vi "Parse Controls Log.vi"(8 "error in (no error)":errorcluster, 11 "Controls Log File":path) -> (0 "error out":errorcluster, 3 "Parsed Pulse Data":T1(array[cluster]))   [LabVIEW 2013, in "Controls Log Monitor.lvlib"]
uses:
  ControlLogParserStateMachineStates.ctl
  PulseData.lvclass
  <vilib>/Utility/miscctls.llb/LVDateTimeRec.ctl
  <vilib>/Utility/file.llb/Read From Spreadsheet File (string).vi
  Controls Log Monitor.lvlib
panel:
  out "Line After Comment":string
  out "Pulse Data Cluster":T2
  out "Entry Index":i32
  out "Pulse Count":i32
  out "Run #":i32
  out "size(s)":i32[](array[numeric])
  out "all rows":string[][](array[string])
  # "68625"
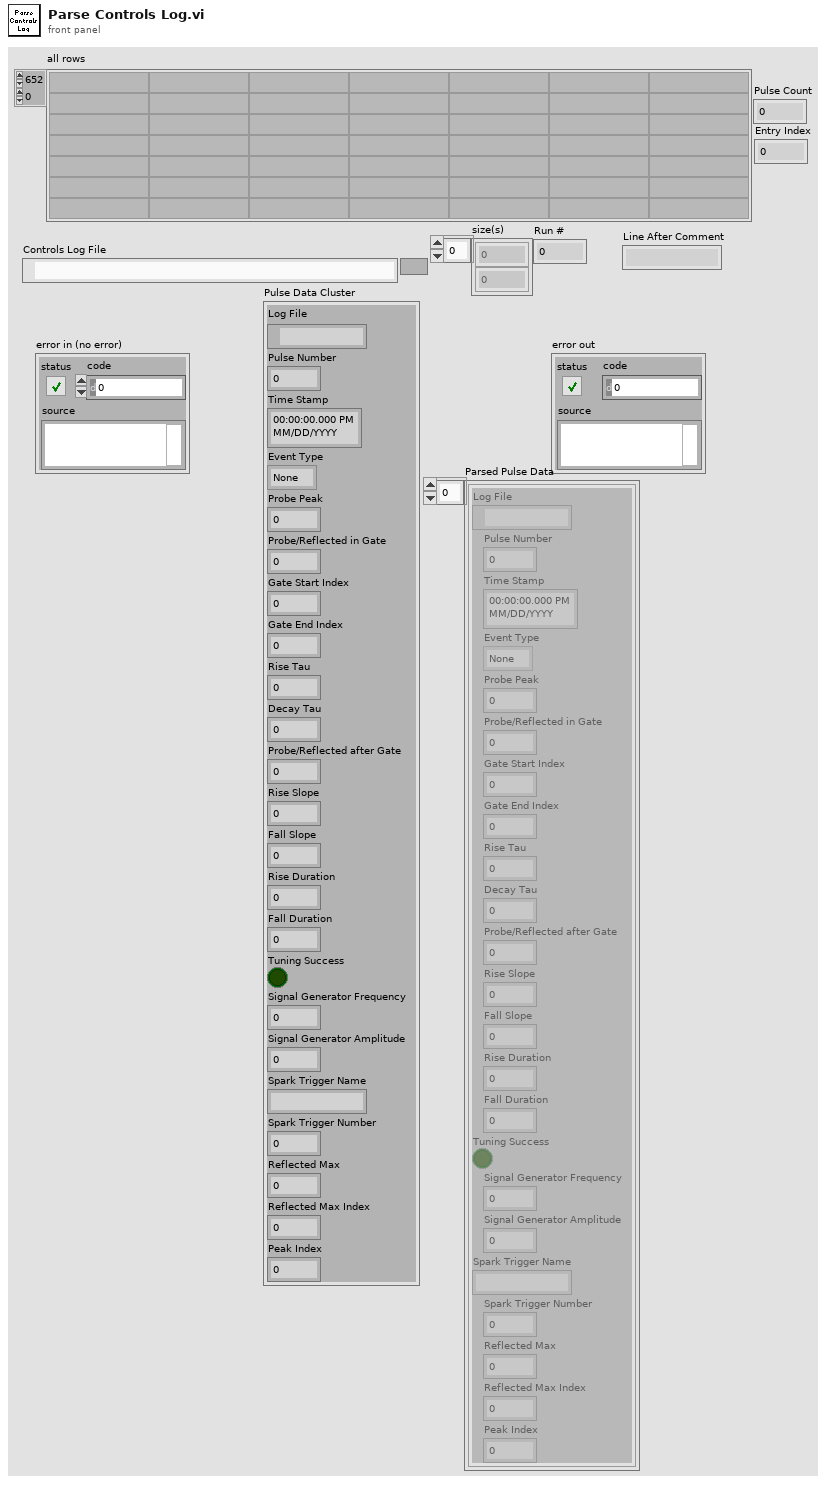
[diagram p1: front panel]
types:
  T1 = cluster{"Log File":path, "Pulse Number":u32, "Time Stamp":timestamp, "Event Type":enum16{"None", "Tune", "Periodic Capture", "Spark Trigger"}, "Probe Peak":dbl, "Probe/Reflected in Gate":dbl, "Gate Start Index":i32, "Gate End Index":i32, "Rise Tau":dbl, "Decay Tau":dbl, "Probe/Reflected after Gate":dbl, "Rise Slope":dbl, "Fall Slope":dbl, "Rise Duration":dbl, "Fall Duration":dbl, "Tuning Success":bool, "Signal Generator Frequency":dbl, "Signal Generator Amplitude":dbl, "Spark Trigger Name":string, "Spark Trigger Number":i32, "Reflected Max":dbl, "Reflected Max Index":i32, "Peak Index":i32}[]
  T2 = cluster{"Log File":path, "Pulse Number":u32, "Time Stamp":timestamp, "Event Type":enum16{"None", "Tune", "Periodic Capture", "Spark Trigger"}, "Probe Peak":dbl, "Probe/Reflected in Gate":dbl, "Gate Start Index":i32, "Gate End Index":i32, "Rise Tau":dbl, "Decay Tau":dbl, "Probe/Reflected after Gate":dbl, "Rise Slope":dbl, "Fall Slope":dbl, "Rise Duration":dbl, "Fall Duration":dbl, "Tuning Success":bool, "Signal Generator Frequency":dbl, "Signal Generator Amplitude":dbl, "Spark Trigger Name":string, "Spark Trigger Number":i32, "Reflected Max":dbl, "Reflected Max Index":i32, "Peak Index":i32}
  T3 = typedef "ControlLogParserStateMachineStates.ctl" = enum16{"Load Log", "Initialize Pulse", "Parse Pulse", "Parse Comment", "Finalize Pulse", "Stop", ""}
  T4 = typedef "LVDateTimeRec.ctl" = cluster{"fractional second":dbl, "second":i32, "minute":i32, "hour":i32, "day of month":i32, "month":i32, "year":i32, "day of week":i32, "day of year":i32, "DST":i32}
  T5 = enum16{"None", "Tune", "Periodic Capture", "Spark Trigger"}
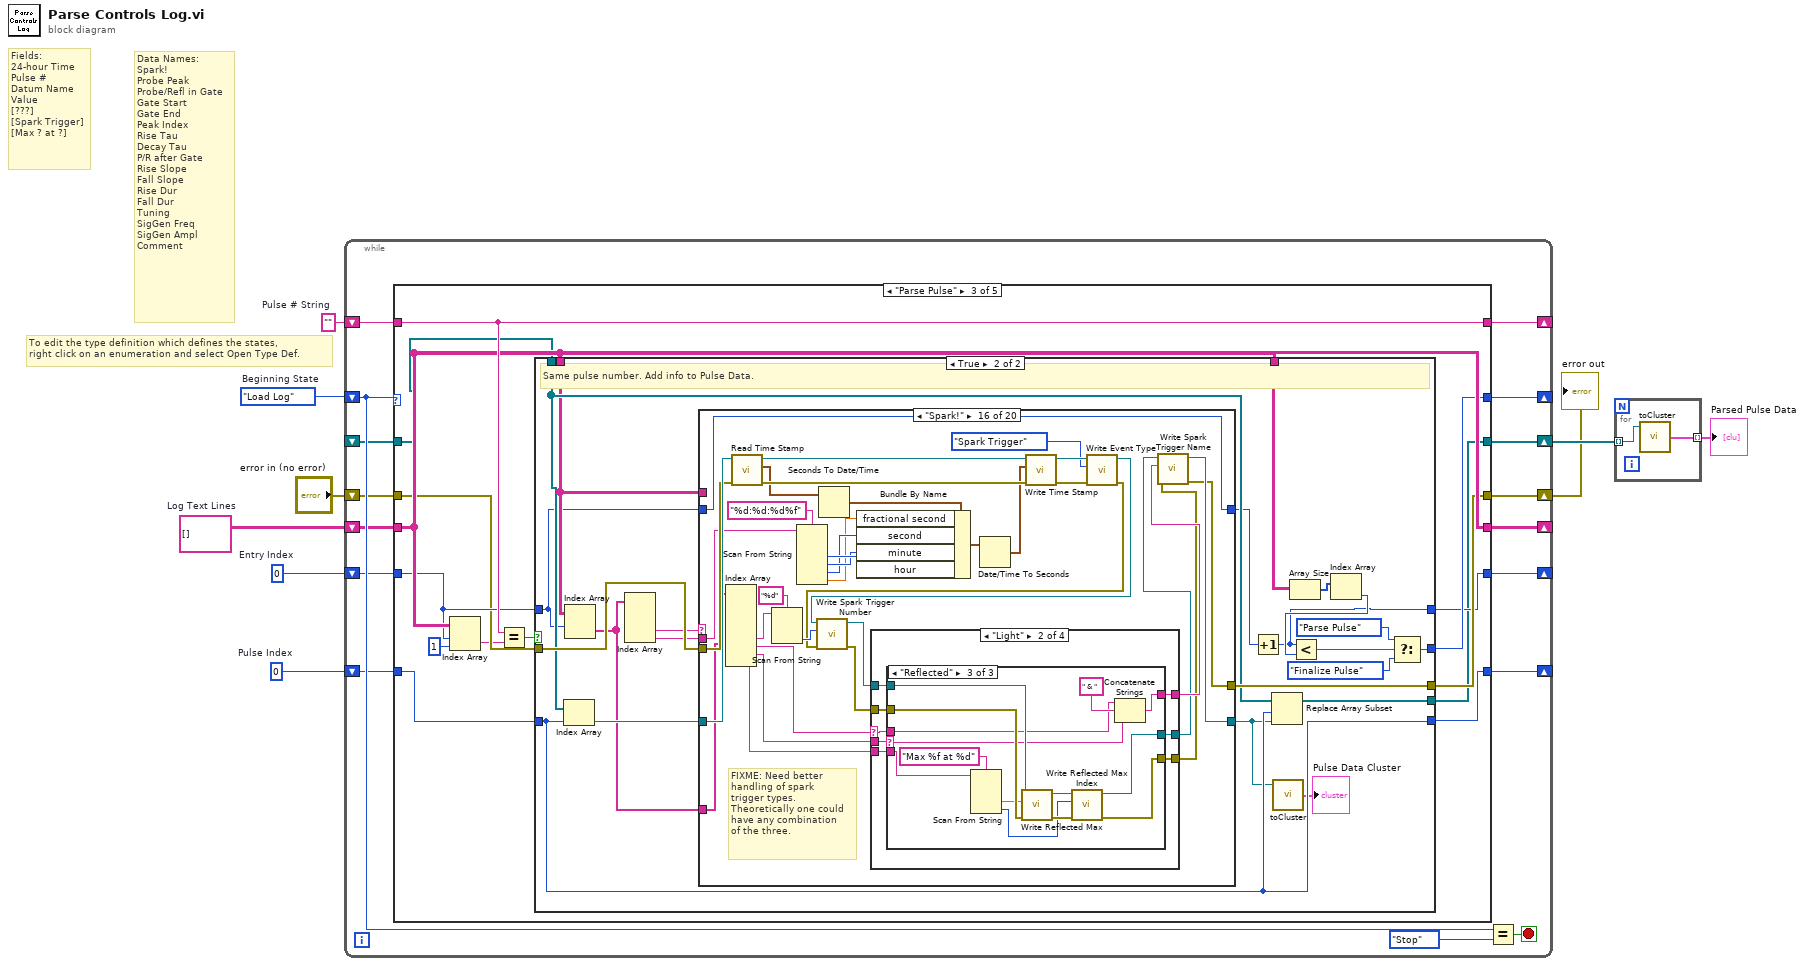
[diagram p0: block diagram]
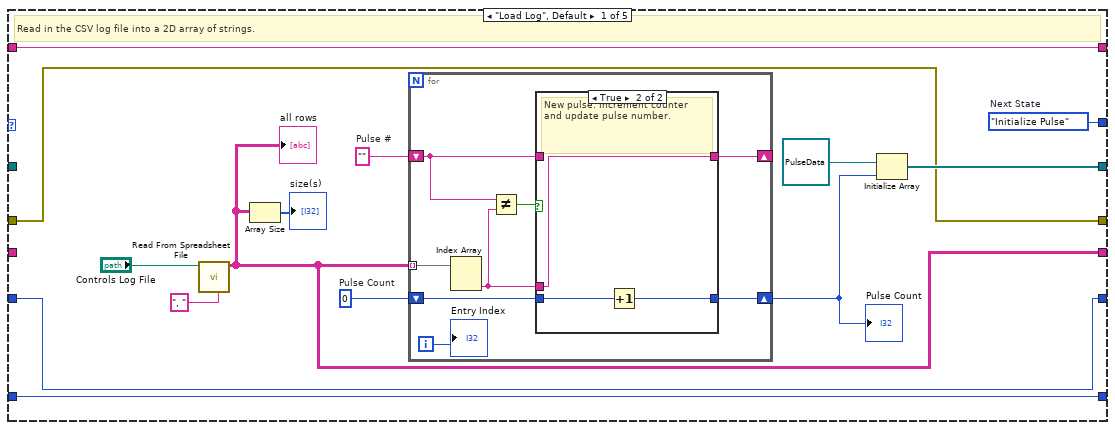
[diagram p2: hidden frame]
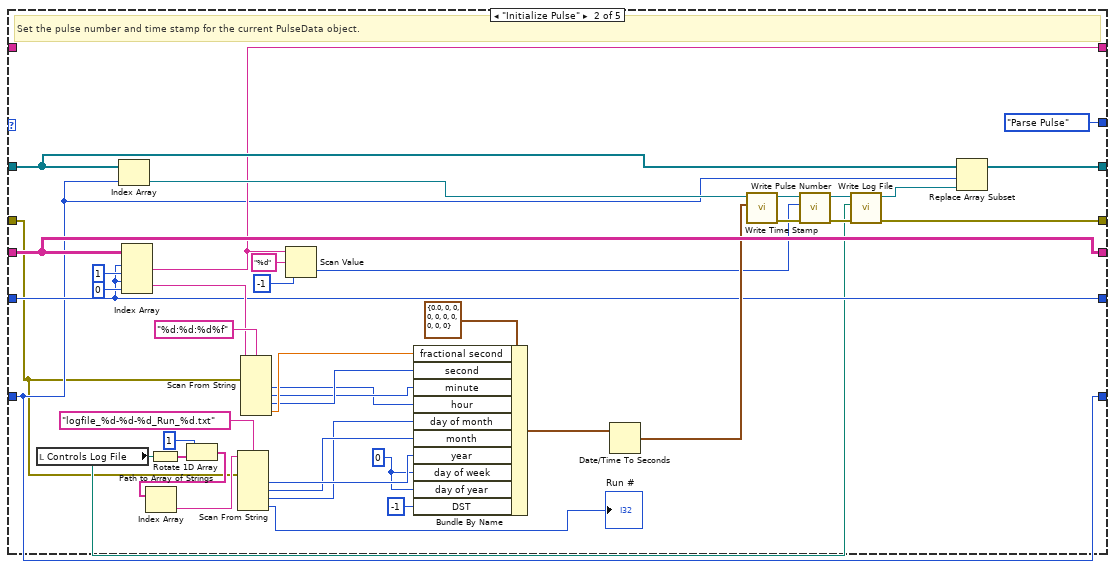
[diagram p4: hidden frame]
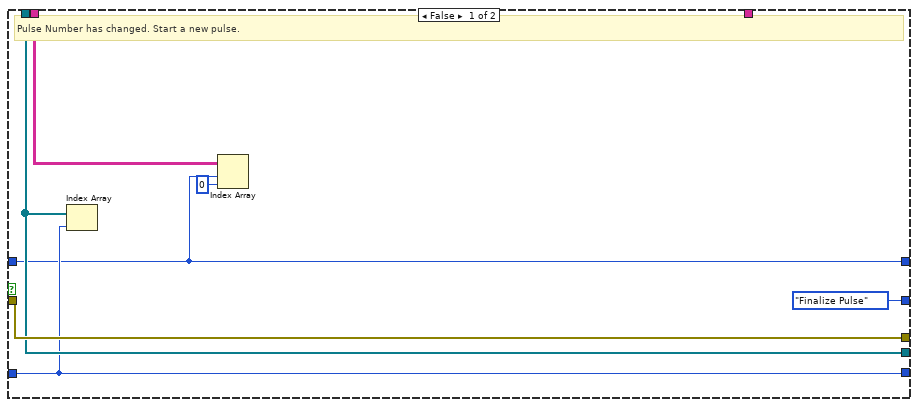
[diagram p5: hidden frame]
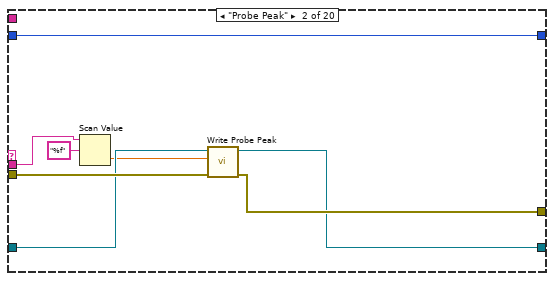
[diagram p7: hidden frame]
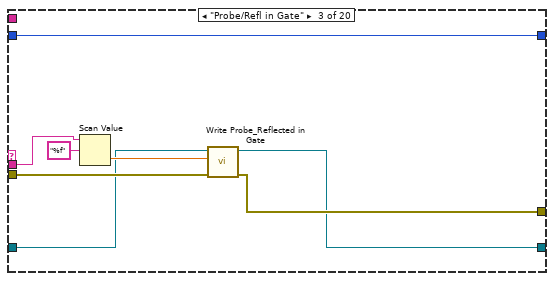
[diagram p8: hidden frame]
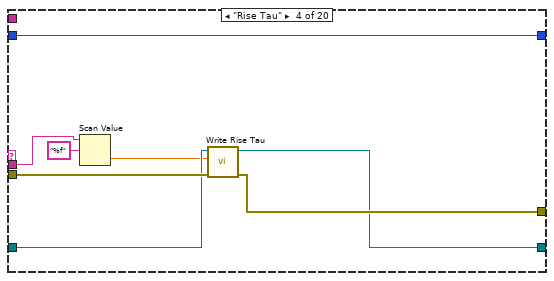
[diagram p9: hidden frame]
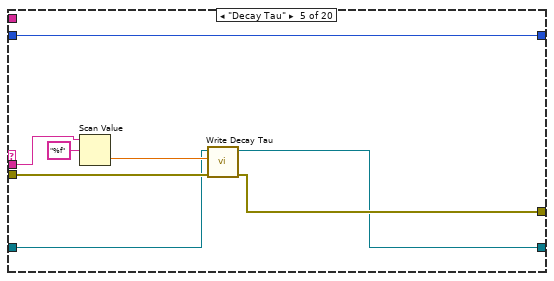
[diagram p10: hidden frame]
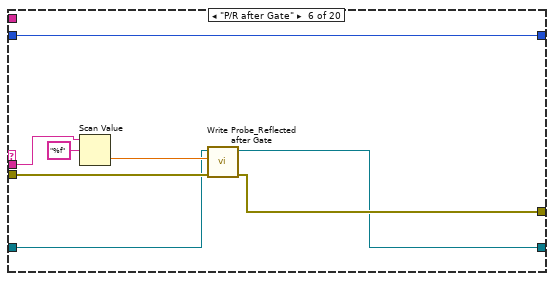
[diagram p11: hidden frame]
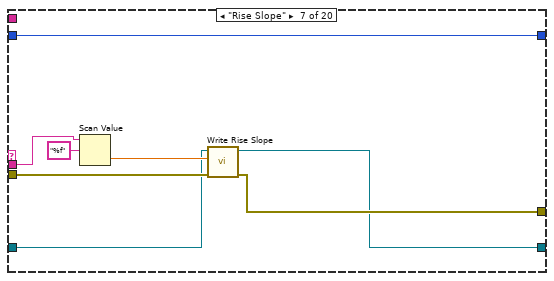
[diagram p12: hidden frame]
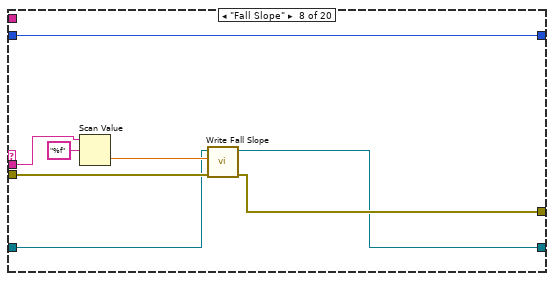
[diagram p13: hidden frame]
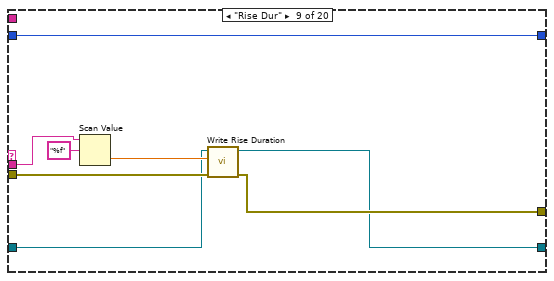
[diagram p14: hidden frame]
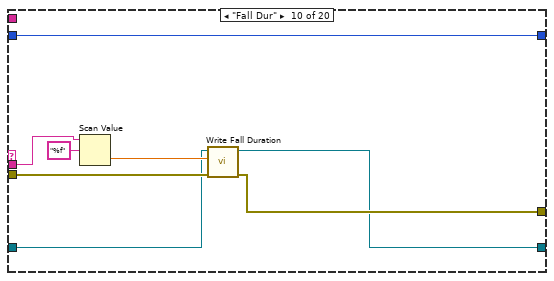
[diagram p15: hidden frame]
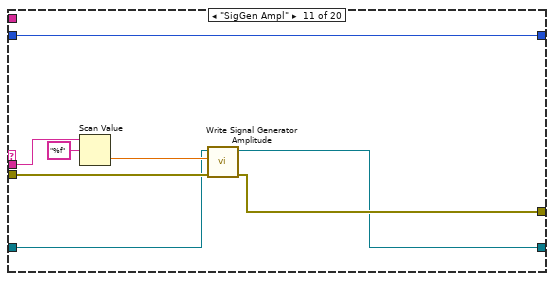
[diagram p16: hidden frame]
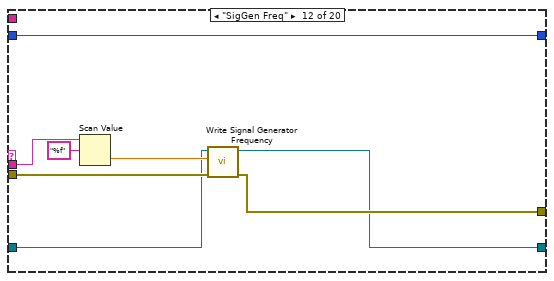
[diagram p17: hidden frame]
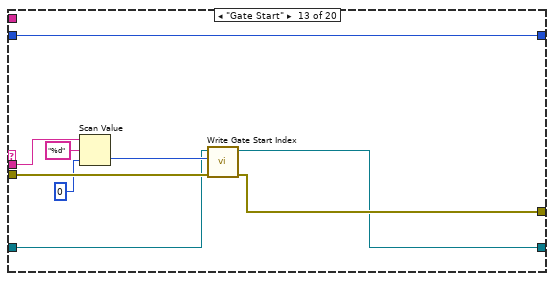
[diagram p18: hidden frame]
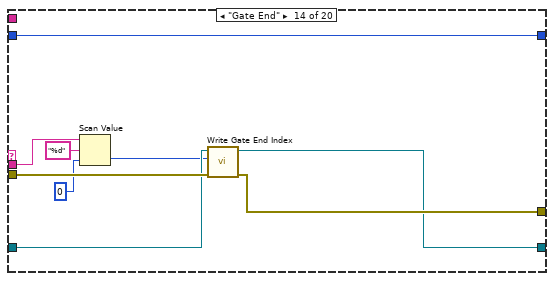
[diagram p19: hidden frame]
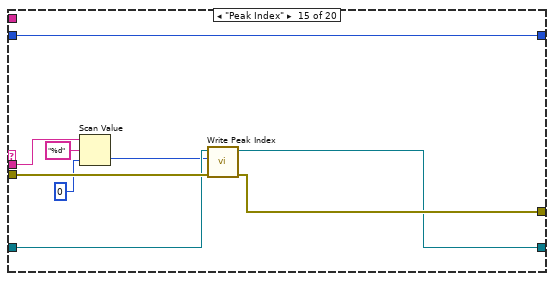
[diagram p20: hidden frame]
diagram:
  w1 = string[][] []  # Log Text Lines
  w5 = ""  # Pulse # String
  w6 = u32 0  # Pulse Index
  w8 = 0  # Entry Index
  w9 = ControlLogParserStateMachineStates."Load Log"  # Beginning State
  # "To edit the type definition which defines the states,\nright click on an enumeration and select Open Type Def."
  # "Data Names:\nSpark!\nProbe Peak\nProbe/Refl in Gate\nGate Start\nGate End\nPeak Index\nRise Tau\nDecay Tau\nP/R after Gate\nRise Slope\nFall Slope\nRise Dur\nFall Dur\nTuning\nSigGen Freq\nSigGen Ampl\nComment"
  # "Fields:\n24-hour Time\nPulse #\nDatum Name\nValue\n[???]\n[Spark Trigger]\n[Max ? at ?]"
  n1 = while {
    shift-right: [w23] -> _
    shift-left: w9 -> [w24]
    shift-right: [w21] -> _
    shift-left: w8 -> [w20]
    shift-right: [w19] -> _
    shift-left: w1 -> [w17]
    shift-right: [w18] -> w4
    shift-left: _ -> [w16]
    shift-right: [w14] -> w3
    shift-left: "error in (no error)" -> [w15]
    shift-right: [w13] -> _
    shift-left: w5 -> [w12]
    shift-right: [w10] -> _
    shift-left: w6 -> [w11]
    stop <- w25 stop-if-true
    n2 = case shown="\"Parse Pulse\"" w24 {
      tunnel: [w39 ControlLogParserStateMachineStates."Parse Pulse" ("Next State") w102 w393 ControlLogParserStateMachineStates."Stop" ("Next State")] -> w23
      tunnel: [w29 w60 w98 w398 w450] -> w21
      tunnel: w20 -> [w29 w60 w103 w398 w450]
      tunnel: [w33 w90 w104 w396 w449] -> w19
      tunnel: [w31 w91 w94 w392 w447] -> w18
      tunnel: w17 -> [_ w90 w104 w396 w449]
      tunnel: w16 -> [_ w92 w101 w391 w447]
      tunnel: w15 -> [w30 w53 w100 w388 w448]
      tunnel: [w30 w55 w99 w389 w448] -> w14
      tunnel: [w28 w61 w106 w402 w446] -> w13
      tunnel: w12 -> [w28 _ w106 w402 w446]
      tunnel: w11 -> [w27 w59 w97 w390 w445]
      tunnel: [w27 w59 w95 w394 w445] -> w10
      frame "Load Log", Default {
        w34 = ""  # Pulse #
        w35 = 0  # Pulse Count
        w39 = ControlLogParserStateMachineStates."Initialize Pulse"  # Next State
        # "Read in the CSV log file into a 2D array of strings."
        n3 = call-poly <vilib>:"Read From Spreadsheet File.vi"("delimiter (\\t)"=", " ("delimiter (\\t)"), "file path (dialog if empty)"="Controls Log File") -> ("all rows"=w33:string[][])  [unwired: 5 in, 4 out]
        "all rows" <- w33
        n4 = Array Size(array=w33) -> (size(s)=→"size(s)":i32[])
        n5 = for {
          tunnel: w33 -> [w47] mode=indexing
          shift-right: [w44] -> w32
          shift-left: w35 -> [w45]
          shift-right: [w42] -> _
          shift-left: w34 -> [w43]
          i -> [w40]
          n6 = Index Array(array=w47) -> (element #2=w41:string)  [unwired: 2 in, 1 out]
          n7 = Not Equal?(x=w43, y=w41) -> (x != y?=w46:bool)
          n8 = case shown="True" w46 {
            tunnel: w45 -> [w49 w52]
            tunnel: [w49 w51] -> w44
            tunnel: w43 -> [w48 _]
            tunnel: [w48 w50] -> w42
            tunnel: w41 -> [_ w50]
            frame False {
            }
            frame True {
              # "New pulse. Increment counter\nand update pulse number."
              n9 = Increment(x=w52) -> (x+1=w51:i32)
            }
          }
          "Entry Index" <- w40
        }
        "Pulse Count" <- w32
        n10 = Initialize Array(refnum<class "PulseData.lvclass"> refnum ("PulseData.lvclass"), w32) -> (w31:refnum<class "PulseData.lvclass">[])
      }
      frame "Initialize Pulse" {
        w75 = 0 ("day of week")
        # "Set the pulse number and time stamp for the current PulseData object."
        n11 = local read "Controls Log File"() -> (w54:path)
        n12 = Index Array(array=w92, index=w59) -> (element=w67:refnum<class "PulseData.lvclass">)
        n13 = Index Array(array=w90, index (row) #1=w60, index (col) #1=1 ("disabled index (col)"), index (row) #2=w60, index (col) #2=0 ("disabled index (col)")) -> (element #1=w61:string, element #2=w85:string)
        n14 = Path to Array of Strings(0:w54) -> (2:w72:string[])  [unwired: 1 out]
        n15 = Rotate 1D Array(1:w72, 2:1 ("n")) -> (0:w70:string[])
        n16 = Index Array(array=w70) -> (element=w69:string)  [unwired: 1 in]
        n17 = Scan From String(format string="logfile_%d-%d-%d_Run_%d.txt", input string=w69, error in=w53) -> (output 1=w79:i32, output 2=w78:i32, output 3=w77:i32, output 4=→"Run #":i32)  [unwired: 5 in, 3 out]
        n18 = Scan From String(format string="%d:%d:%d%f", input string=w85, error in=w53) -> (output 1=w80:i32, output 2=w81:i32, output 3=w82:i32, output 4=w83:dbl)  [unwired: 5 in, 3 out]
        n19 = Scan Value(string=w61, format string="%d", default (0 dbl)=-1) -> (value=w62:i32)  [unwired: 1 out]
        n20 = Bundle By Name(cluster=T4 {"fractional second"=0.0, "second"=0, "minute"=0, "hour"=0, "day of month"=0, "month"=0, "year"=0, "day of week"=0, "day of year"=0, "DST"=0} ("date time rec"), "fractional second"=w83, "second"=w82, "minute"=w81, "hour"=w80, "day of month"=w77, "month"=w78, "year"=w79, "day of week"=w75, "day of year"=w75, "DST"=-1) -> (w74:T4)
        n21 = Date/Time To Seconds(2:w74) -> (0:w68:timestamp)  [unwired: 1 in]
        n22 = call-dynamic "Write Time Stamp.vi"("Time Stamp"=w68, "PulseData in"=w67) -> ("error out"=w65:errorcluster, "PulseData out"=w66:refnum<class "PulseData.lvclass">)  [unwired: 8 in]
        n23 = call-dynamic "Write Pulse Number.vi"("error in (no error)"=w65, "Pulse Number"=w62, "PulseData in"=w66) -> ("error out"=w57:errorcluster, "PulseData out"=w58:refnum<class "PulseData.lvclass">)  [unwired: 7 in]
        n24 = call-dynamic "Write Log File.vi"("error in (no error)"=w57, "Log File"=w54, "PulseData in"=w58) -> ("error out"=w55:errorcluster, "PulseData out"=w56:refnum<class "PulseData.lvclass">)  [unwired: 7 in]
        n25 = Replace Array Subset(array=w92, new element=w56, index=w59) -> (w91:refnum<class "PulseData.lvclass">[])
      }
      frame "Parse Pulse" {
        n26 = Index Array(array=w104, index (row)=w103, index (col)=1) -> (element=w96:string)
        n27 = Equal?(x=w106, y=w96) -> (x = y?=w105:bool)
        n28 = case shown="True" w105 {
          tunnel: w104 -> [w108 w117]
          tunnel: w103 -> [w110 w116]
          tunnel: w104 -> [_ w136]
          tunnel: [ControlLogParserStateMachineStates."Finalize Pulse" ("Next State") w130] -> w102
          tunnel: w101 -> [w112 w125]
          tunnel: w100 -> [w113 w129]
          tunnel: [w113 w128] -> w99
          tunnel: [w110 w127] -> w98
          tunnel: w97 -> [w111 w120]
          tunnel: [w111 w120] -> w95
          tunnel: [w112 w124] -> w94
          frame False {
            # "Pulse Number has changed. Start a new pulse."
            n29 = Index Array(array=w112, index=w111) -> ()  [unwired: 1 out]
            n30 = Index Array(array=w108, index (row)=w110, index (col)=0) -> ()  [unwired: 1 out]
          }
          frame True {
            # "Same pulse number. Add info to Pulse Data."
            n31 = Index Array(array=w125, index=w120) -> (element=w126:refnum<class "PulseData.lvclass">)
            n32 = Index Array(array=w117, index (row)=w116) -> (element=w121:string[])  [unwired: 1 in]
            n33 = Index Array(array=w121) -> (element #3=w123:string, element #4=w122:string)  [unwired: 4 in, 2 out]
            n34 = case shown="\"Spark!\"" w123 {
              tunnel: w129 -> [w139 w146 w153 w162 w170 w178 w186 w194 w202 w210 w218 w226 w235 w245 w254 w285 w338 w349 w365 w371]
              tunnel: [w139 w145 w152 w161 w169 w177 w185 w193 w201 w209 w217 w225 w234 w244 w253 w264 w337 w351 w365 w371] -> w128
              tunnel: w122 -> [_ w144 w151 w160 w168 w176 w184 w192 w200 w208 w216 w224 w233 w239 w248 w275 _ w353 _ _]
              tunnel: w126 -> [w138 w143 w150 w159 w166 w174 w182 w190 w198 w206 w214 w222 w230 w243 w252 w288 w339 w348 w364 w370]
              tunnel: [w138 w142 w149 w157 w165 w173 w181 w189 w197 w205 w213 w221 w229 w242 w251 w265 w335 w350 w364 w370] -> w119
              tunnel: w121 -> [_ _ _ _ _ _ _ _ _ _ _ _ _ _ _ w271 _ _ _ _]
              tunnel: w117 -> [_ _ _ _ _ _ _ _ _ _ _ _ _ _ _ _ _ _ _ w369]
              tunnel: w116 -> [w137 w140 w148 w156 w164 w172 w180 w188 w196 w204 w212 w220 w228 w237 w246 w255 w334 w340 w363 w368]
              tunnel: [w137 w140 w148 w156 w164 w172 w180 w188 w196 w204 w212 w220 w228 w237 w246 w255 w334 w340 w363 w367] -> w115
              frame Default {
              }
              frame "Probe Peak" {
                n35 = Scan Value(string=w144, format string="%f") -> (value=w141:dbl)  [unwired: 1 in, 1 out]
                n36 = call-dynamic "Write Probe Peak.vi"("error in (no error)"=w146, "Probe Peak"=w141, "PulseData in"=w143) -> ("error out"=w145:errorcluster, "PulseData out"=w142:refnum<class "PulseData.lvclass">)  [unwired: 7 in]
              }
              frame "Probe/Refl in Gate" {
                n37 = Scan Value(string=w151, format string="%f") -> (value=w154:dbl)  [unwired: 1 in, 1 out]
                n38 = call-dynamic "Write Probe_Reflected in Gate.vi"("error in (no error)"=w153, "Probe/Reflected in Gate"=w154, "PulseData in"=w150) -> ("error out"=w152:errorcluster, "PulseData out"=w149:refnum<class "PulseData.lvclass">)  [unwired: 7 in]
              }
              frame "Rise Tau" {
                n39 = Scan Value(string=w160, format string="%f") -> (value=w158:dbl)  [unwired: 1 in, 1 out]
                n40 = call-dynamic "Write Rise Tau.vi"("error in (no error)"=w162, "Rise Tau"=w158, "PulseData in"=w159) -> ("error out"=w161:errorcluster, "PulseData out"=w157:refnum<class "PulseData.lvclass">)  [unwired: 7 in]
              }
              frame "Decay Tau" {
                n41 = Scan Value(string=w168, format string="%f") -> (value=w167:dbl)  [unwired: 1 in, 1 out]
                n42 = call-dynamic "Write Decay Tau.vi"("error in (no error)"=w170, "Decay Tau"=w167, "PulseData in"=w166) -> ("error out"=w169:errorcluster, "PulseData out"=w165:refnum<class "PulseData.lvclass">)  [unwired: 7 in]
              }
              frame "P/R after Gate" {
                n43 = Scan Value(string=w176, format string="%f") -> (value=w175:dbl)  [unwired: 1 in, 1 out]
                n44 = call-dynamic "Write Probe_Reflected after Gate.vi"("error in (no error)"=w178, "Probe/Reflected after Gate"=w175, "PulseData in"=w174) -> ("error out"=w177:errorcluster, "PulseData out"=w173:refnum<class "PulseData.lvclass">)  [unwired: 7 in]
              }
              frame "Rise Slope" {
                n45 = Scan Value(string=w184, format string="%f") -> (value=w183:dbl)  [unwired: 1 in, 1 out]
                n46 = call-dynamic "Write Rise Slope.vi"("error in (no error)"=w186, "Rise Slope"=w183, "PulseData in"=w182) -> ("error out"=w185:errorcluster, "PulseData out"=w181:refnum<class "PulseData.lvclass">)  [unwired: 7 in]
              }
              frame "Fall Slope" {
                n47 = Scan Value(string=w192, format string="%f") -> (value=w191:dbl)  [unwired: 1 in, 1 out]
                n48 = call-dynamic "Write Fall Slope.vi"("error in (no error)"=w194, "Fall Slope"=w191, "PulseData in"=w190) -> ("error out"=w193:errorcluster, "PulseData out"=w189:refnum<class "PulseData.lvclass">)  [unwired: 7 in]
              }
              frame "Rise Dur" {
                n49 = Scan Value(string=w200, format string="%f") -> (value=w199:dbl)  [unwired: 1 in, 1 out]
                n50 = call-dynamic "Write Rise Duration.vi"("error in (no error)"=w202, "Rise Duration"=w199, "PulseData in"=w198) -> ("error out"=w201:errorcluster, "PulseData out"=w197:refnum<class "PulseData.lvclass">)  [unwired: 7 in]
              }
              frame "Fall Dur" {
                n51 = Scan Value(string=w208, format string="%f") -> (value=w207:dbl)  [unwired: 1 in, 1 out]
                n52 = call-dynamic "Write Fall Duration.vi"("error in (no error)"=w210, "Fall Duration"=w207, "PulseData in"=w206) -> ("error out"=w209:errorcluster, "PulseData out"=w205:refnum<class "PulseData.lvclass">)  [unwired: 7 in]
              }
              frame "SigGen Ampl" {
                n53 = Scan Value(string=w216, format string="%f") -> (value=w215:dbl)  [unwired: 1 in, 1 out]
                n54 = call-dynamic "Write Signal Generator Amplitude.vi"("error in (no error)"=w218, "Signal Generator Amplitude"=w215, "PulseData in"=w214) -> ("error out"=w217:errorcluster, "PulseData out"=w213:refnum<class "PulseData.lvclass">)  [unwired: 7 in]
              }
              frame "SigGen Freq" {
                n55 = Scan Value(string=w224, format string="%f") -> (value=w223:dbl)  [unwired: 1 in, 1 out]
                n56 = call-dynamic "Write Signal Generator Frequency.vi"("error in (no error)"=w226, "Signal Generator Frequency"=w223, "PulseData in"=w222) -> ("error out"=w225:errorcluster, "PulseData out"=w221:refnum<class "PulseData.lvclass">)  [unwired: 7 in]
              }
              frame "Gate Start" {
                n57 = Scan Value(string=w233, format string="%d", default (0 dbl)=u32 0) -> (value=w231:u32)  [unwired: 1 out]
                n58 = call-dynamic "Write Gate Start Index.vi"("error in (no error)"=w235, "Gate Start Index"=w231, "PulseData in"=w230) -> ("error out"=w234:errorcluster, "PulseData out"=w229:refnum<class "PulseData.lvclass">)  [unwired: 7 in]
              }
              frame "Gate End" {
                n59 = Scan Value(string=w239, format string="%d", default (0 dbl)=u32 0) -> (value=w238:u32)  [unwired: 1 out]
                n60 = call-dynamic "Write Gate End Index.vi"("error in (no error)"=w245, "Gate End Index"=w238, "PulseData in"=w243) -> ("error out"=w244:errorcluster, "PulseData out"=w242:refnum<class "PulseData.lvclass">)  [unwired: 7 in]
              }
              frame "Peak Index" {
                n61 = Scan Value(string=w248, format string="%d", default (0 dbl)=u32 0) -> (value=w247:u32)  [unwired: 1 out]
                n62 = call-dynamic "Write Peak Index.vi"("error in (no error)"=w254, "Peak Index"=w247, "PulseData in"=w252) -> ("error out"=w253:errorcluster, "PulseData out"=w251:refnum<class "PulseData.lvclass">)  [unwired: 7 in]
              }
              frame "Spark!" {
                # "FIXME: Need better\nhandling of spark\ntrigger types.\nTheoretically one could\nhave any combination\nof the three."
                n63 = Index Array(array=w271) -> (element #5=w274:string, element #6=w256:string, element #7=w258:string, element #8=w257:string)  [unwired: 8 in, 4 out]
                n64 = call-dynamic "Read Time Stamp.vi"("error in (no error)"=w285, "PulseData in"=w288) -> ("error out"=w286:errorcluster, "Time Stamp"=w284:timestamp, "PulseData out"=w287:refnum<class "PulseData.lvclass">)  [unwired: 7 in]
                n65 = Scan From String(format string="%d", input string=w274) -> (output 1=w272:i32)  [unwired: 3 in, 3 out]
                n66 = Scan From String(format string="%d:%d:%d%f", input string=w275) -> (output 1=w281:i32, output 2=w280:i32, output 3=w279:i32, output 4=w278:dbl)  [unwired: 6 in, 3 out]
                n67 = Seconds To Date/Time(time stamp (now)=w284) -> (date time rec=w283:T4)  [unwired: 1 in]
                n68 = Bundle By Name(cluster=w283, "fractional second"=w278, "second"=w279, "minute"=w280, "hour"=w281) -> (w277:T4)
                n69 = Date/Time To Seconds(2:w277) -> (0:w276:timestamp)  [unwired: 1 in]
                n70 = call-dynamic "Write Time Stamp.vi"("error in (no error)"=w286, "Time Stamp"=w276, "PulseData in"=w287) -> ("error out"=w262:errorcluster, "PulseData out"=w263:refnum<class "PulseData.lvclass">)  [unwired: 7 in]
                n71 = call-dynamic "Write Event Type.vi"("error in (no error)"=w262, "Event Type"=T5."Spark Trigger", "PulseData in"=w263) -> ("error out"=w260:errorcluster, "PulseData out"=w261:refnum<class "PulseData.lvclass">)  [unwired: 7 in]
                n72 = call-dynamic "Write Spark Trigger Number.vi"("error in (no error)"=w260, "Spark Trigger Index"=w272, "PulseData in"=w261) -> ("error out"=w269:errorcluster, "PulseData out"=w270:refnum<class "PulseData.lvclass">)  [unwired: 7 in]
                n73 = case shown="\"Light\"" w256 {
                  selector: w256 -> [_ w293 w321 w333]
                  tunnel: w270 -> [w291 w299 w324 w332]
                  tunnel: w269 -> [w289 w298 w325 w331]
                  tunnel: ["" ("String") w297 w321 w333] -> w268
                  tunnel: [w289 w296 w323 w331] -> w267
                  tunnel: [w291 w295 w322 w332] -> w266
                  tunnel: w258 -> [_ w292 w320 _]
                  tunnel: w257 -> [_ w294 _ _]
                  frame Default {
                  }
                  frame "Light" {
                    n74 = case shown="\"Reflected\"" w292 {
                      selector: w292 -> [_ _ w306]
                      tunnel: ["" ("String") w303 w311] -> w297
                      tunnel: w299 -> [w301 w305 w318]
                      tunnel: w298 -> [w300 w304 w317]
                      tunnel: [w300 w304 w310] -> w296
                      tunnel: [w301 w305 w309] -> w295
                      tunnel: w293 -> [_ w303 w308]
                      tunnel: w294 -> [_ _ w307]
                      frame Default {
                      }
                      frame "" {
                      }
                      frame "Reflected" {
                        n75 = Scan From String(format string="Max %f at %d", input string=w307) -> (output 1=w316:dbl, output 2=w313:i32)  [unwired: 4 in, 3 out]
                        n76 = call-dynamic "Write Reflected Max.vi"("error in (no error)"=w317, "Reflected Max Something"=w316, "PulseData in"=w318) -> ("error out"=w314:errorcluster, "PulseData out"=w315:refnum<class "PulseData.lvclass">)  [unwired: 7 in]
                        n77 = call-dynamic "Write Reflected Max Index.vi"("error in (no error)"=w314, "Reflected Max Index"=w313, "PulseData in"=w315) -> ("error out"=w310:errorcluster, "PulseData out"=w309:refnum<class "PulseData.lvclass">)  [unwired: 7 in]
                        n78 = Concatenate Strings(w308, " & " ("string"), w306) -> (w311:string)
                      }
                    }
                  }
                  frame "Reflected" {
                    n79 = Scan From String(format string="Max %f at %d", input string=w320) -> (output 1=w329:dbl, output 2=w326:i32)  [unwired: 4 in, 3 out]
                    n80 = call-dynamic "Write Reflected Max.vi"("error in (no error)"=w325, "Reflected Max Something"=w329, "PulseData in"=w324) -> ("error out"=w327:errorcluster, "PulseData out"=w328:refnum<class "PulseData.lvclass">)  [unwired: 7 in]
                    n81 = call-dynamic "Write Reflected Max Index.vi"("error in (no error)"=w327, "Reflected Max Index"=w326, "PulseData in"=w328) -> ("error out"=w323:errorcluster, "PulseData out"=w322:refnum<class "PulseData.lvclass">)  [unwired: 7 in]
                  }
                  frame "Duration" {
                  }
                }
                n82 = call-dynamic "Write Spark Trigger Name.vi"("error in (no error)"=w267, "Spark Trigger Name"=w268, "PulseData in"=w266) -> ("error out"=w264:errorcluster, "PulseData out"=w265:refnum<class "PulseData.lvclass">)  [unwired: 7 in]
              }
              frame "Periodic Capture" {
                n83 = call-dynamic "Write Event Type.vi"("error in (no error)"=w338, "Event Type"=T5."Periodic Capture", "PulseData in"=w339) -> ("error out"=w337:errorcluster, "PulseData out"=w335:refnum<class "PulseData.lvclass">)  [unwired: 7 in]
              }
              frame "Tuning" {
                # "Tunning events can happen on any pulse. If there is no event type\nassigned yet, set it to Tune. It may get changed later, but that's ok."
                n84 = call-dynamic "Read Event Type.vi"("error in (no error)"=w349, "PulseData in"=w348) -> ("error out"=w344:errorcluster, "Event Type"=w346:T5, "PulseData out"=w343:refnum<class "PulseData.lvclass">)  [unwired: 7 in]
                n85 = Equal?(x=w346, y=T5."None" ("Event Type")) -> (x = y?=w345:bool)
                n86 = case shown="True" w345 {
                  tunnel: w344 -> [w354 w359]
                  tunnel: w343 -> [w355 w358]
                  tunnel: [w355 w357] -> w341
                  tunnel: [w354 w356] -> w342
                  frame False {
                  }
                  frame True {
                    n87 = call-dynamic "Write Event Type.vi"("error in (no error)"=w359, "Event Type"=T5."Tune", "PulseData in"=w358) -> ("error out"=w356:errorcluster, "PulseData out"=w357:refnum<class "PulseData.lvclass">)  [unwired: 7 in]
                  }
                }
                n88 = case shown="\"Success\"" w353 {
                  tunnel: [FALSE TRUE] -> w352
                  frame "Failed", Default {
                  }
                  frame "Success" {
                  }
                }
                n89 = call-dynamic "Write Tuning Success.vi"("error in (no error)"=w342, "Tuning Success"=w352, "PulseData in"=w341) -> ("error out"=w351:errorcluster, "PulseData out"=w350:refnum<class "PulseData.lvclass">)  [unwired: 7 in]
              }
              frame "Ampl Mon start", "Run Number", "Starting 201 MHz NI-Scope Waveforms -DWP.vi", "Target Ampl (dBm)" {
              }
              frame "Comment" {
                n90 = while {
                  tunnel: w369 -> [w377]
                  shift-right: [w372] -> w366
                  shift-left: w368 -> [w375]
                  stop <- w376 continue-if-true
                  # "Multiline comments will\nhave lines that don't parse\nproperly. Skip them."
                  n91 = Increment(x=w375) -> (x+1=w372:i32)
                  n92 = Index Array(array=w377, index (row)=w372, index (col)=0 ("disabled index (col)")) -> (element=w373:string)
                  "Line After Comment" <- w373
                  n93 = Scan From String(format string="%d:%d:%d%f", input string=w373) -> (error out=w376:errorcluster)  [unwired: 10 in, 2 out]
                }
                n94 = Decrement(x=w366) -> (x-1=w367:i32)
              }
            }
            n95 = Increment(x=w115) -> (x+1=w127:i32)
            n96 = Replace Array Subset(array=w125, new element=w119, index=w120) -> (w124:refnum<class "PulseData.lvclass">[])
            n97 = call-dynamic "toCluster.vi"("PulseData in"=w119) -> ("Pulse Data Cluster"=→"Pulse Data Cluster":T2)  [unwired: 2 in, 2 out]
            n98 = Array Size(array=w136) -> (size(s)=w135:i32[])
            n99 = Index Array(array=w135) -> (element=w134:i32)  [unwired: 1 in]
            n100 = Less?(x=w127, y=w134) -> (x < y?=w133:bool)
            n101 = Select(t=ControlLogParserStateMachineStates."Parse Pulse" ("Next State"), s=w133, f=ControlLogParserStateMachineStates."Finalize Pulse" ("Next State")) -> (s? t:f=w130:T3)
          }
        }
      }
      frame "Finalize Pulse" {
        n102 = Index Array(array=w391, index=w390) -> (element=w387:refnum<class "PulseData.lvclass">)
        n103 = Array Size(array=w396) -> (size(s)=w397:i32[])
        n104 = Index Array(array=w397) -> (element=w395:i32)  [unwired: 1 in]
        n105 = call-dynamic "Read Event Type.vi"("error in (no error)"=w388, "PulseData in"=w387) -> ("error out"=w386:errorcluster, "Event Type"=w382:T5, "PulseData out"=w384:refnum<class "PulseData.lvclass">)  [unwired: 7 in]
        n106 = Less?(x=w398, y=w395) -> (x < y?=w401:bool)
        n107 = Equal?(x=w382, y=T5."None" ("Event Type")) -> (x = y?=w383:bool)
        n108 = Select(t=ControlLogParserStateMachineStates."Initialize Pulse" ("Next State"), s=w401, f=ControlLogParserStateMachineStates."Stop" ("Next State")) -> (s? t:f=w393:T3)
        n109 = case shown="True" w383 {
          tunnel: w386 -> [w405 w412]
          tunnel: w384 -> [w403 w411]
          tunnel: [w405 w413] -> w385
          tunnel: [FALSE w409] -> _
          tunnel: [w403 w406] -> w380
          frame False {
          }
          frame True {
            n110 = call-dynamic "toCluster.vi"("error in (no error)"=w412, "PulseData in"=w411) -> ("error out"=w413:errorcluster, "Pulse Data Cluster"=w434:T2, "PulseData out"=w406:refnum<class "PulseData.lvclass">)  [unwired: 1 in]
            n111 = Unbundle By Name(w434) -> ("Pulse Number"=w414:u32, "Probe Peak"=w433:dbl, "Probe/Reflected in Gate"=w432:dbl, "Gate Start Index"=w424:i32, "Gate End Index"=w423:i32, "Rise Tau"=w431:dbl, "Probe/Reflected after Gate"=w430:dbl, "Rise Slope"=w429:dbl, "Fall Slope"=w428:dbl, "Rise Duration"=w427:dbl, "Fall Duration"=w426:dbl, "Signal Generator Frequency"=w418:dbl, "Signal Generator Amplitude"=w417:dbl, "Spark Trigger Number"=w422:i32, "Reflected Max"=w425:dbl, "Reflected Max Index"=w421:i32)  [unwired: 4 out]
            n112 = Build Array(w414, w424, w423, w422, w421) -> (w419:u32[])
            n113 = Build Array(w433, w432, w431, w430, w429, w428, w427, w426, w418, w417, w425) -> (w420:dbl[])
            n114 = Build Array(w418, w417) -> (w408:dbl[])
            n115 = Add Array Elements(numeric array=w408) -> (sum=w407:dbl)
            n116 = Add Array Elements(numeric array=w420) -> (sum=w416:dbl)
            n117 = Add Array Elements(numeric array=w419) -> (sum=w415:u32)
            n118 = Add(x=w416, y=w415) -> (x+y=w410:dbl)
            n119 = Equal?(x=w410, y=w407) -> (x = y?=w409:bool)
          }
        }
        n120 = case shown="True" FALSE {
          tunnel: w391 -> [w436 w443]
          tunnel: w390 -> [_ w441]
          tunnel: w385 -> [w435 w444]
          tunnel: [w436 w440] -> w392
          tunnel: w380 -> [_ w439]
          tunnel: [w435 w438] -> w389
          frame False {
          }
          frame True {
            n121 = call-dynamic "Write Event Type.vi"("error in (no error)"=w444, "Event Type"=T5."Tune", "PulseData in"=w439) -> ("error out"=w438:errorcluster, "PulseData out"=w442:refnum<class "PulseData.lvclass">)  [unwired: 7 in]
            n122 = Replace Array Subset(array=w443, new element=w442, index=w441) -> (w440:refnum<class "PulseData.lvclass">[])
          }
        }
        n123 = Increment(x=w390) -> (x+1=w394:u32)
      }
      frame "Stop" {
      }
    }
    n124 = Equal?(x=w24, y=ControlLogParserStateMachineStates."Stop" ("Stop")) -> (x = y?=w25:bool)
  }
  "error out" <- w3
  n125 = for {
    tunnel: w4 -> [w453] mode=indexing
    tunnel: [w452] -> w2 mode=indexing
    n126 = call-dynamic "toCluster.vi"("PulseData in"=w453) -> ("Pulse Data Cluster"=w452:T2)  [unwired: 2 in, 2 out]
  }
  "Parsed Pulse Data" <- w2
